vi "VeriStand DSF.Transfer.Configuration.Verify.No Buffer Overlaps.vi"(8 "error in (no error)":errorcluster, 11 "channel configurations":T1[](array[typedef]) {"count" format="%d bytes"}) -> (0 "error out":errorcluster)   [LabVIEW 2017, in "Data Sharing Custom Device Engine.lvlib" / "VeriStand DSF.Transfer.Configuration.lvclass"]
uses:
  VeriStand DSF.Transfer.Configuration.lvclass
  Builds/Data Sharing Framework/Current/Data Sharing Framework Core/DSF Core.lvlibp/DSF Configuration API/Public/Controls/DSF Engine Channel Configuration.ctl
  Builds/Data Sharing Framework/Current/Data Sharing Framework Core/DSF Core.lvlibp/DSF Configuration API/Public/Controls/DSF Data Type.ctl
  Builds/Data Sharing Framework/Current/Data Sharing Framework Core/DSF Core.lvlibp/DSF Configuration API/Public/Controls/DSF Settings Info.ctl
  Builds/Data Sharing Framework/Current/Data Sharing Framework Core/DSF Core.lvlibp
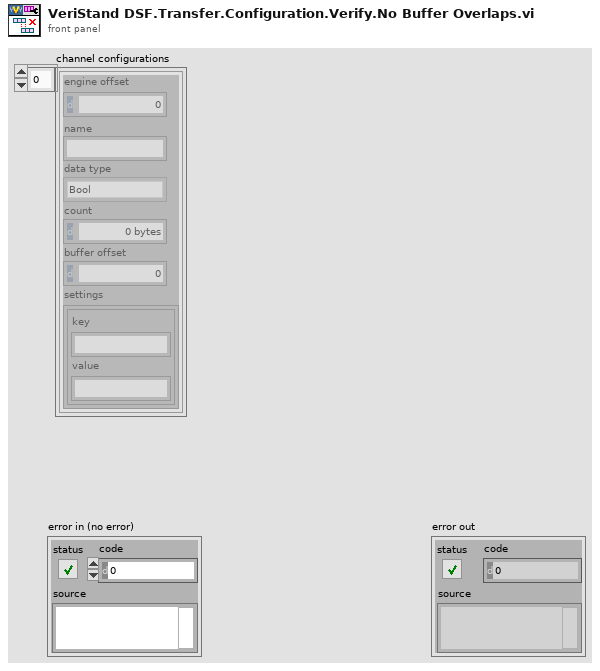
[diagram p1: front panel]
types:
  T1 = typedef "DSF Core.lvlibp/DSF Engine Channel Configuration.ctl" = cluster{"engine offset":u64, "name":string, "data type":T2, "count":u64, "buffer offset":u64, "settings":T3}
  T2 = typedef "DSF Core.lvlibp/DSF Data Type.ctl" = enum8{"Bool", "SGL", "DBL", "I8", "I16", "I32", "I64", "U8", "U16", "U32", "U64"}
  T3 = typedef "DSF Core.lvlibp/DSF Settings Info.ctl" = cluster{"key":string, "value":string}[]
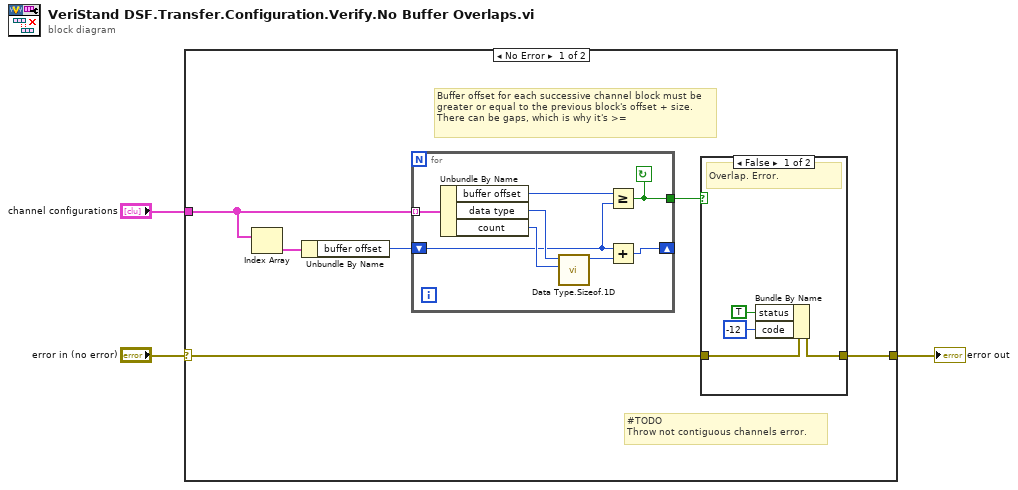
[diagram p0: block diagram]
diagram:
  n1 = case shown="No Error" "error in (no error)" {
    selector: "error in (no error)" -> [w4 w23]
    tunnel: "channel configurations" -> [w9 _]
    tunnel: [w5 w23] -> w2
    frame No Error {
      # "#TODO\nThrow not contiguous channels error."
      # "Buffer offset for each successive channel block must be greater or equal to the previous block's offset + size. There can be gaps, which is why it's >="
      n2 = Index Array(array=w9) -> (element=w7:T1)  [unwired: 1 in]
      n3 = Unbundle By Name(w7) -> ("buffer offset"=w8:u64)
      n4 = for {
        shift-right: [w14] -> _
        shift-left: w8 -> [w10]
        tunnel: w9 -> [w17] mode=indexing
        tunnel: [w15] -> w6
        stop <- w15 continue-if-true
        n5 = Unbundle By Name(w17) -> ("buffer offset"=w16:u64, "data type"=w11:T2, "count"=w12:u64)
        n6 = call "Data Type.Sizeof.1D.vi"("count"=w12, "data type"=w11) -> ("size in bytes"=w13:u64)  [unwired: 9 in]
        n7 = Greater Or Equal?(x=w16, y=w10) -> (x >= y?=w15:bool)
        n8 = Add(x=w10, y=w13) -> (x+y=w14:u64)
      }
      n9 = case shown="False" w6 {
        tunnel: w4 -> [w21 w22]
        tunnel: [w18 w22] -> w5
        frame False {
          # "Overlap. Error."
          n10 = Bundle By Name(cluster=w21, "status"=TRUE, "code"=-12) -> (w18:errorcluster)
        }
        frame True {
          # "No overlaps. Proceed."
        }
      }
    }
    frame Error {
    }
  }
  "error out" <- w2
